vi "DiscArchiver.change file.vi"(0 "i ref in":refnum<vi>, 3 "ms timeout (10000)":i32=10000, 5 "error in (no error)":errorcluster) -> (14 "i ref out":refnum<vi>, 17 "timed out":bool, 19 "error out":errorcluster)   [LabVIEW 2014, in "DiscArchiver.lvlib"]
doc: "Closes the actual (old) file and opens a new file."
uses:
  DiscArchiver.lvlib
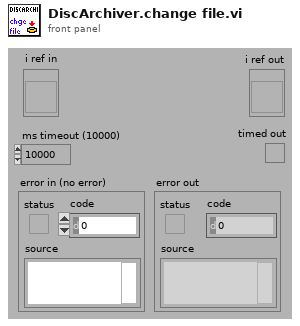
[diagram p1: front panel]
types:
  T1 = typedef "DiscArchiver.lvlib/DiscArchiver.i attribute.ctl" = cluster{"file prefix":string, "actual file":string, "nOfEvents":i32, "file":refnum<file>, "eventBuilder":string, "disc size alarm":bool, "dataDescription":string, "dataDescriptionURL":string, "eventDataURL":string, "headerID":dbl, "completeData":bool, "nOfEventsID":i32, "dataFileID":i32}
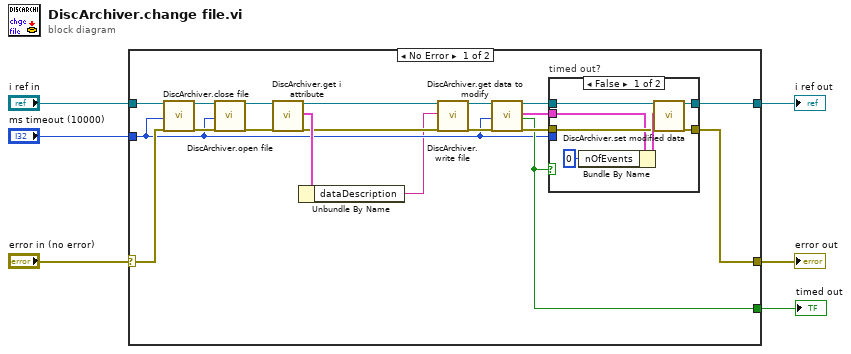
[diagram p0: block diagram]
diagram:
  n1 = case shown="No Error" "error in (no error)" {
    selector: "error in (no error)" -> [w12 w35]
    tunnel: [w25 w36] -> w6
    tunnel: "i ref in" -> [w21 w36]
    tunnel: "ms timeout (10000)" -> [w8 _]
    tunnel: [w13 w35] -> w3
    tunnel: [w11 _] -> w1
    frame No Error {
      n2 = call "DiscArchiver.close file.vi"("i ref in"=w21, "ms timeout (10000)"=w8, "error in (no error)"=w12) -> ("i ref out"=w20:refnum<vi>, "error out"=w19:errorcluster)  [unwired: 14 in, 1 out]
      n3 = call "DiscArchiver.open file.vi"("i ref in"=w20, "ms timeout (10000)"=w8, "error in (no error)"=w19) -> ("i ref out"=w18:refnum<vi>, "error out"=w17:errorcluster)  [unwired: 14 in, 1 out]
      n4 = call "DiscArchiver.get i attribute.vi"("i ref in"=w18, "error in (no error)"=w17) -> ("i ref out"=w10:refnum<vi>, "i attribute"=w16:T1, "error out"=w9:errorcluster)  [unwired: 15 in]
      n5 = Unbundle By Name(w16) -> ("dataDescription"=w7:string)
      n6 = call "DiscArchiver.write file.vi"("i ref in"=w10, "eventData"=w7, "error in (no error)"=w9) -> ("i ref out"=w15:refnum<vi>, "error out"=w14:errorcluster)  [unwired: 15 in]
      n7 = call "DiscArchiver.get data to modify.vi"("i ref in"=w15, "ms timeout (10000)"=w8, "error in (no error)"=w14) -> ("i ref out"=w24:refnum<vi>, "i attribute"=w22:T1, "timed out"=w11:bool, "error out"=w23:errorcluster)  [unwired: 13 in]
      n8 = case "timed out?" shown="False" w11 {
        tunnel: [w32 w33] -> w13
        tunnel: [w31 w34] -> w25
        tunnel: w24 -> [w29 w34]
        tunnel: w23 -> [w27 w33]
        tunnel: w22 -> [w26 _]
        tunnel: w8 -> [_ _]
        frame False {
          n9 = Bundle By Name(cluster=w26, "nOfEvents"=0 ("# of items")) -> (w30:T1)
          n10 = call "DiscArchiver.set modified data.vi"("i ref in"=w29, "i attribute"=w30, "error in (no error)"=w27) -> ("i ref out"=w31:refnum<vi>, "error out"=w32:errorcluster)  [unwired: 15 in]
        }
        frame True {
        }
      }
    }
    frame Error {
    }
  }
  "error out" <- w3
  "i ref out" <- w6
  "timed out" <- w1
